vi "Lab0_Select.vi"() -> ()   [LabVIEW 2014]
panel:
  out "Output":string
  in  "Click This!":bool
  in  "stop":bool
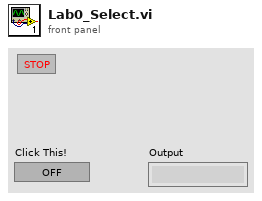
[diagram p1: front panel]
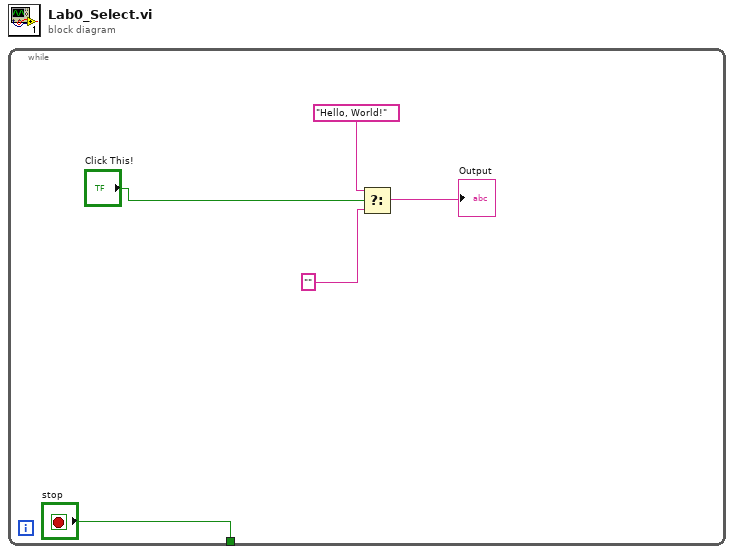
[diagram p0: block diagram]
diagram:
  n1 = while {
    tunnel: ["stop"] -> _
    stop <- "stop" stop-if-true
    n2 = Select(t="Hello, World!", s="Click This!", f="") -> (s? t:f=→"Output":string)
  }
